vi "XIPIN_AXI_Crossbar_2_1.vi"   [LabVIEW 2017]
doc: "The AXI Crossbar IP provides the infrastructure to connect multiple AXI4/AXI3/AXI4-Lite masters and slaves.\n------------------------------------\n<b>Need License</b> : No\n<b>Interface</b> : AXI4"
uses:
  <vilib>/rvi/XilinxIP/XIPIN_XNode/niFpgaXIPIN.xnode
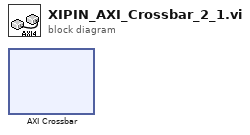
[diagram p0: block diagram]
diagram:
  n1 = xnode ("AXI Crossbar")() -> ()
